vi "CalcRatiosBouncer.vi"(9 "Run Summary":T2 {"C12LE" format="%_3e"; "C13LE" format="%_3e"; "C1312" format="%_3e"; "C12" format="%_3e"; "C13L" format="%_3e"; "C13H" format="%_3e"}) -> (1 "Run Ratios":T1 {"LEC13/12" format="%_4e"; "DTfrac" format="%#_3g"; "DT" format="%#_3g"; "CountErr" format="%#_3g"; "d13C" format="%_4g"; "C13/12" format="%_4e"; "C14/12" format="%_4e"; "C14/13" format="%_3e"; "C12Cor" format="%_3e"; "C13" format="%_3e"; "C13H/L" format="%#_3g"})   [LabVIEW 2013]
uses:
  ctl/SummaryData.ctl
  ctl/RunRatios.ctl
panel:
  in  "Run Ratios In":T1 {"LEC13/12" format="%_4e"; "DTfrac" format="%#_3g"; "DT" format="%#_3g"; "CountErr" format="%#_3g"; "d13C" format="%_4g"; "C13/12" format="%_4e"; "C14/12" format="%_4e"; "C14/13" format="%_3e"; "C12Cor" format="%_3e"; "C13" format="%_3e"; "C13H/L" format="%#_3g"}
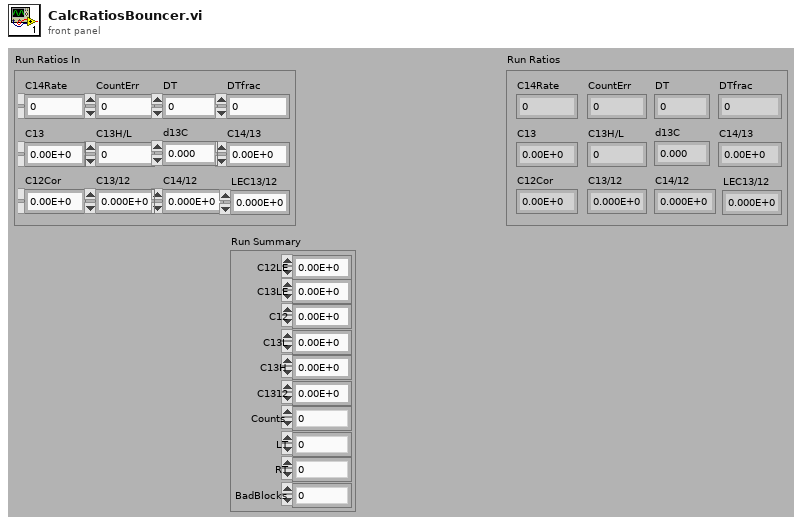
[diagram p1: front panel]
types:
  T1 = typedef "RunRatios.ctl" = cluster{"C14Rate":dbl, "CountErr":dbl, "DT":dbl, "DTfrac":dbl, "C13":dbl, "C13H/L":dbl, "d13C":dbl, "C14/13":dbl, "C12Cor":dbl, "C13/12":dbl, "C14/12":dbl, "LEC13/12":dbl}
  T2 = typedef "SummaryData.ctl" = cluster{"C12LE":dbl, "C13LE":dbl, "C12":dbl, "C13L":dbl, "C13H":dbl, "C1312":dbl, "Counts":u32, "LT":dbl, "RT":dbl, "BadBlocks":u8}
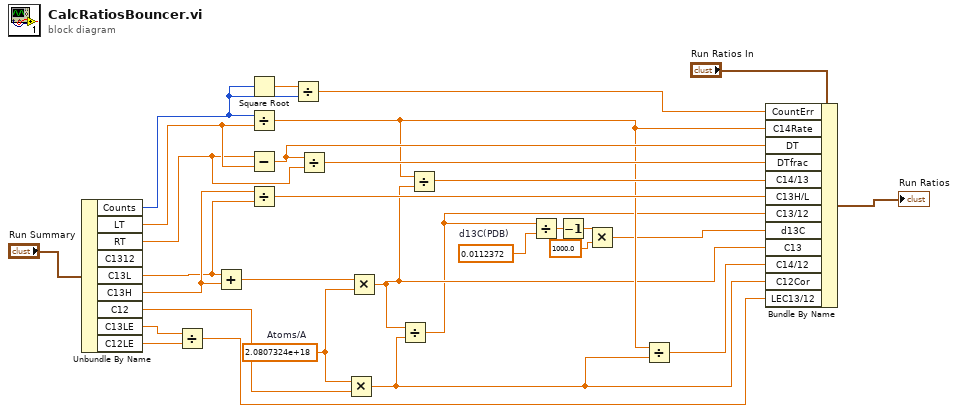
[diagram p0: block diagram]
diagram:
  w25 = 0.0112372  # d13C(PDB)
  w24 = 2.0807324e+18  # Atoms/A
  n1 = Unbundle By Name("Run Summary") -> ("Counts"=w19:u32, "LT"=w22:dbl, "RT"=w21:dbl, "C13L"=w8:dbl, "C13H"=w20:dbl, "C12"=w7:dbl, "C13LE"=w6:dbl, "C12LE"=w5:dbl)  [unwired: 1 out]
  n2 = Divide(x=w6, y=w5) -> (x/y=w4:dbl)
  n3 = Add(x=w8, y=w20) -> (x+y=w30:dbl)
  n4 = Square Root(x=w19) -> (sqrt(x)=w29:dbl)
  n5 = Divide(x=w19, y=w22) -> (x/y=w12:dbl)
  n6 = Subtract(x=w21, y=w22) -> (x-y=w16:dbl)
  n7 = Divide(x=w20, y=w8) -> (x/y=w13:dbl)
  n8 = Divide(x=w29, y=w19) -> (x/y=w11:dbl)
  n9 = Divide(x=w16, y=w21) -> (x/y=w15:dbl)
  n10 = Multiply(x=w24, y=w7) -> (x*y=w2:dbl)
  n11 = Multiply(x=w30, y=w24) -> (x*y=w3:dbl)
  n12 = Divide(x=w3, y=w2) -> (x/y=w1:dbl)
  n13 = Divide(x=w12, y=w3) -> (x/y=w14:dbl)
  n14 = Divide(x=w1, y=w25) -> (x/y=w27:dbl)
  n15 = Decrement(x=w27) -> (x-1=w28:dbl)
  n16 = Multiply(x=w28, y=1000.0) -> (x*y=w9:dbl)
  n17 = Divide(x=w12, y=w2) -> (x/y=w10:dbl)
  n18 = Bundle By Name(cluster="Run Ratios In", "CountErr"=w11, "C14Rate"=w12, "DT"=w16, "DTfrac"=w15, "C14/13"=w14, "C13H/L"=w13, "C13/12"=w1, "d13C"=w9, "C13"=w3, "C14/12"=w10, "C12Cor"=w2, "LEC13/12"=w4) -> (→"Run Ratios":T1)
